vi "Create identity matrix.vi"(5 "Matrix size":i32) -> (2 "Identity Matrix":T1)   [LabVIEW 2016]
uses:
  <vilib>/Analysis/Matrix/Datatypes/ComplexMatrix.ctl
  <vilib>/Analysis/Matrix/Numeric/Conversions/Array To Matrix - CA2.vi
  <vilib>/Analysis/Matrix/NI_Matrix.lvlib
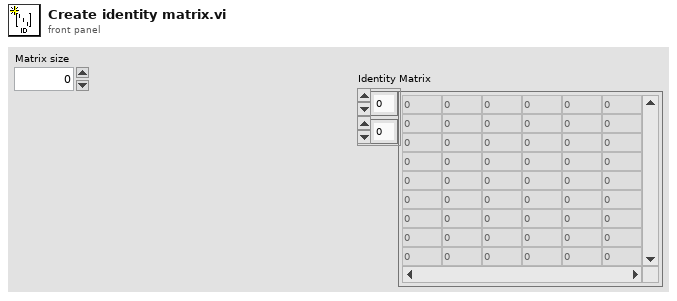
[diagram p1: front panel]
types:
  T1 = typedef "NI_Matrix.lvlib/ComplexMatrix.ctl" = cdb[][]
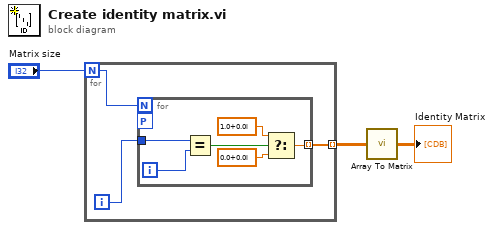
[diagram p0: block diagram]
diagram:
  n1 = for {
    N: "Matrix size" -> [w6]
    tunnel: [w4] -> w2 mode=indexing
    i -> [w5]
    n2 = for {
      N: w6 -> [_]
      tunnel: w5 -> [w10]
      tunnel: [w7] -> w4 mode=indexing
      workers-P: _ -> [_]
      i -> [w9]
      n3 = Equal?(x=w10, y=w9) -> (x = y?=w8:bool)
      n4 = Select(t=cdb 1.0+0.0i ("Complex Matrix Element"), s=w8, f=cdb 0.0+0.0i ("Complex Matrix Element")) -> (s? t:f=w7:cdb)
    }
  }
  n5 = call-poly <vilib>:"Array To Matrix.vi"("Complex 2D Array"=w2) -> ("Complex Matrix"=→"Identity Matrix":T1)
